vi "DENEME.vi"() -> ()   [LabVIEW 2018]
uses:
  <vilib>/Instr/_visa.llb/VISA Configure Serial Port (Instr).vi
panel:
  out "read buffer":string
  out "Thermometer":dbl(slide) scale=0.0..100.0
  out "TEMP":i32
  in  "VISA resource name":refnum<visa-resource-name>="COM7"
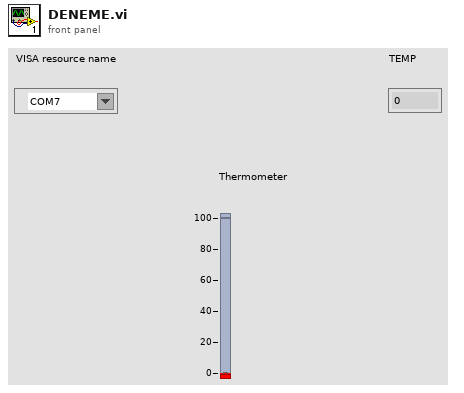
[diagram p1: front panel]
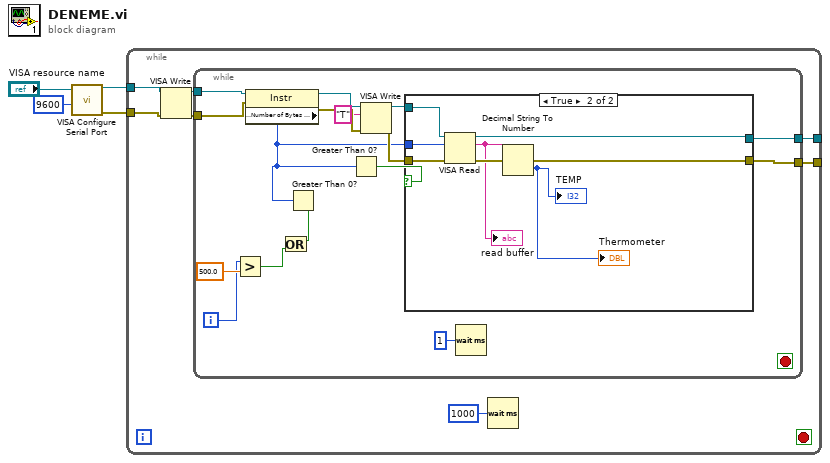
[diagram p0: block diagram]
diagram:
  n1 = call-poly "VISA Configure Serial Port"("VISA resource name"="VISA resource name", "baud rate (9600)"=u32 9600) -> ("VISA resource name out"=w2:refnum<visa-resource-name>, "error out"=w1:errorcluster)  [unwired: 12 in]
  n2 = while {
    tunnel: w2 -> [w11]
    tunnel: w1 -> [w10]
    tunnel: [w6] -> _
    tunnel: [w5] -> _
    stop <- _ stop-if-true
    n3 = VISA Write(VISA resource name=w11, error in (no error)=w10) -> (VISA resource name out=w9:refnum<visa-resource-name>, error out=w8:errorcluster)  [unwired: 1 in, 1 out]
    n4 = while {
      tunnel: w9 -> [w27]
      tunnel: w8 -> [w26]
      tunnel: [w14] -> w6
      tunnel: [w13] -> w5
      i -> [w22]
      stop <- _ stop-if-true
      n5 = Greater?(x=w22, y=500.0) -> (0:w21:bool)
      n6 = property class="Instr"(reference=w27, error in=w26) -> (reference out=w25:refnum<visa-resource-name>, error out=w24:errorcluster, "Serial Settings:Number of Bytes at Serial Port"=w16:u32)
      n7 = Greater Than 0?(x=w16) -> (x > 0?=w20:bool)
      n8 = Or(x=w20, y=w21) -> ()  [unwired: 1 out]
      n9 = Greater Than 0?(x=w16) -> (x > 0?=w19:bool)
      n10 = VISA Write(VISA resource name=w25, write buffer="T", error in (no error)=w24) -> (VISA resource name out=w18:refnum<visa-resource-name>, error out=w17:errorcluster)  [unwired: 1 out]
      n11 = case shown="True" w19 {
        tunnel: w18 -> [_ w34]
        tunnel: w17 -> [_ w33]
        tunnel: w16 -> [_ w32]
        tunnel: [_ w31] -> w14
        tunnel: [_ w30] -> w13
        frame False {
        }
        frame True {
          n12 = VISA Read(VISA resource name=w34, byte count=w32, error in (no error)=w33) -> (VISA resource name out=w31:refnum<visa-resource-name>, read buffer=w28:string, error out=w30:errorcluster)  [unwired: 1 out]
          "read buffer" <- w28
          n13 = Decimal String To Number(string=w28) -> (number=→"TEMP" →"Thermometer":i32)  [unwired: 2 in, 1 out]
        }
      }
      n14 = Wait (ms)(milliseconds to wait=u32 1) -> ()  [unwired: 1 out]
    }
    n15 = Wait (ms)(milliseconds to wait=u32 1000) -> ()  [unwired: 1 out]
  }
